vi "scripting_v4.vi"() -> ()   [LabVIEW 2020]
uses:
  <vilib>/numeric/LVNumericRepresentation.ctl
panel:
  out "appended path":path
  out "concatenated string":string
  out "resulting string":string
  out "error out 2":errorcluster
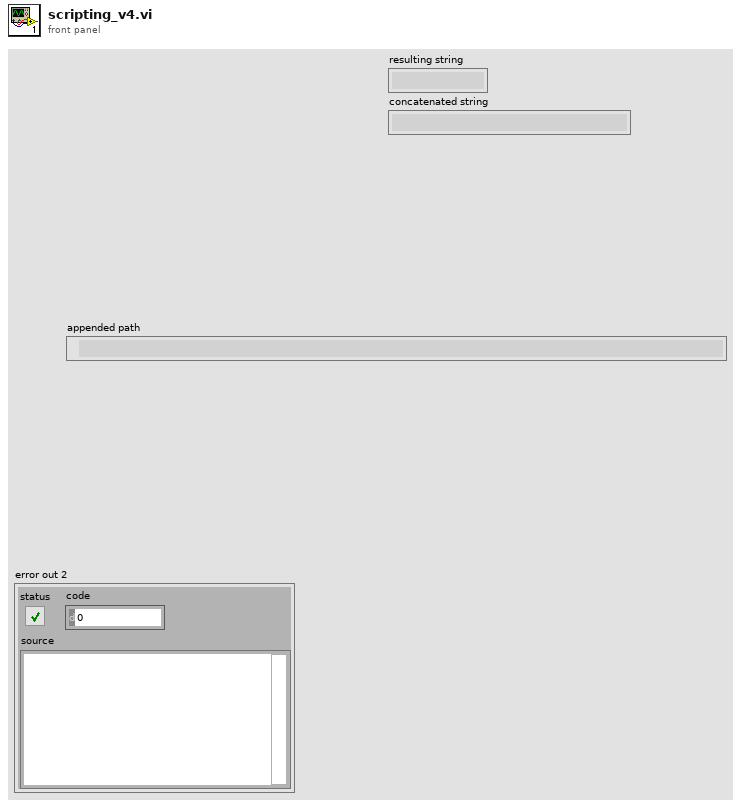
[diagram p1: front panel]
types:
  T1 = typedef "LVNumericRepresentation.ctl" = enum32{"Extended Precision", "Double Precision", "Single Precision", "Long", "Word", "Byte", "Unsigned Long", "Unsigned Word", "Unsigned Byte", "Complex Extended", "Complex Double", "Complex Single", "Quad", "Unsigned Quad", "Fixed-Point"}
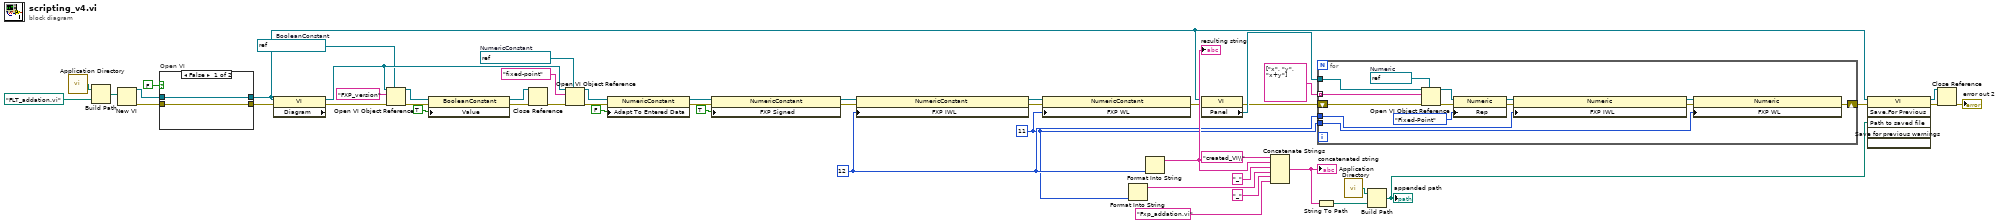
[diagram p0: block diagram]
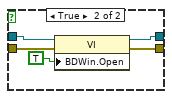
[diagram p2: hidden frame]
diagram:
  w10 = refnum<vi> refnum  # BooleanConstant
  w19 = refnum<vi> refnum  # NumericConstant
  w20 = 11 ("Fixed-Point Representation:Bits:Word Length")
  w21 = 12 ("Fixed-Point Representation:Bits:Integer Word Length")
  n1 = call <vilib>:"Application Directory.vi"() -> ("Application Directory"=w41:path)
  n2 = Build Path(base path=w41, name or relative path=path "FLT_addation.vi" ("vi path")) -> (appended path=w39:path)
  n3 = New VI(10:w39) -> (0:w49:errorcluster, 3:w50:refnum<vi>)  [unwired: 6 in]
  n4 = case "Open VI" shown="False" FALSE {
    tunnel: w50 -> [w51 w57]
    tunnel: w49 -> [w52 w56]
    tunnel: [w51 w54] -> w26
    tunnel: [w52 w53] -> w27
    frame False {
    }
    frame True {
      n5 = property class="VI"(reference=w57, error in=w56, "BDWin.Open"=TRUE ("Block Diagram Window:Open")) -> (reference out=w54:refnum<vi>, error out=w53:errorcluster)
    }
  }
  n6 = property on="Property Node" class="VI" props=["Diagram"](reference=w26, error in=w27) -> (reference out=w11:refnum<vi>, error out=w8:errorcluster)  [unwired: 1 out]
  n7 = Open VI Object Reference(7:w10, 8:w8, 10:"FXP_version" ("name/order"), 11:w11) -> (0:w6:errorcluster, 3:w7:refnum<vi>)
  n8 = property on="Property Node" class="BooleanConstant"(reference=w7, error in=w6, "Value"=TRUE ("Adapt To Entered Data")) -> (reference out=w3:refnum<vi>, error out=w2:errorcluster)
  n9 = Close Reference(reference=w3, error in (no error)=w2) -> (error out=w1:errorcluster)
  n10 = Open VI Object Reference(7:w19, 8:w1, 10:"fixed-point" ("name/order"), 11:w11) -> (0:w9:errorcluster, 3:w15:refnum<vi>)
  n11 = property on="Property Node" class="NumericConstant"(reference=w15, error in=w9, "Adapt To Entered Data"=FALSE) -> (reference out=w14:refnum<vi>, error out=w13:errorcluster)
  n12 = property on="Property Node" class="NumericConstant"(reference=w14, error in=w13, "FXP Signed"=TRUE ("Fixed-Point Representation:Bits:Signed")) -> (reference out=w18:refnum<vi>, error out=w17:errorcluster)
  n13 = property on="Property Node" class="NumericConstant"(reference=w18, error in=w17, "FXP IWL"=w21) -> (reference out=w24:refnum<vi>, error out=w23:errorcluster)
  n14 = property on="Property Node" class="NumericConstant"(reference=w24, error in=w23, "FXP WL"=w20) -> (error out=w22:errorcluster)  [unwired: 1 out]
  n15 = Format Into String(w20) -> (resulting string=w34:string)  [unwired: 3 in, 1 out]
  n16 = Format Into String(w21) -> (resulting string=w36:string)  [unwired: 3 in, 1 out]
  "resulting string" <- w36
  n17 = property on="Property Node" class="VI"(reference=w26, error in=w22) -> (error out=w43:errorcluster, "Panel"=w44:refnum<vi>)  [unwired: 1 out]
  n18 = Concatenate Strings("created_VI\\" ("string"), w36, "_" ("string"), w34, "_" ("string"), "Fxp_addation.vi" ("string")) -> (w32:string)
  "concatenated string" <- w32
  n19 = String To Path(string=w32) -> (path=w30:path)
  n20 = for {
    tunnel: w44 -> [w69]
    tunnel: w21 -> [w60]
    tunnel: w20 -> [w59]
    shift-right: [w61] -> w42
    shift-left: w43 -> [w67]
    tunnel: string[] ["x", "y", "x+y"] -> [w58] mode=indexing
    w71 = refnum<vi> refnum  # Numeric
    n21 = Open VI Object Reference(7:w71, 8:w67, 10:w58, 11:w69) -> (0:w68:errorcluster, 3:w70:refnum<vi>)
    n22 = property on="Property Node" class="Numeric"(reference=w70, error in=w68, "Rep"=LVNumericRepresentation."Fixed-Point" ("new representation")) -> (reference out=w65:refnum<vi>, error out=w64:errorcluster)
    n23 = property on="Property Node" class="Numeric"(reference=w65, error in=w64, "FXP IWL"=w60) -> (reference out=w63:refnum<vi>, error out=w62:errorcluster)
    n24 = property on="Property Node" class="Numeric"(reference=w63, error in=w62, "FXP WL"=w59) -> (error out=w61:errorcluster)  [unwired: 1 out]
  }
  n25 = call <vilib>:"Application Directory.vi"() -> ("Application Directory"=w38:path)
  n26 = Build Path(base path=w38, name or relative path=w30) -> (appended path=w37:path)
  "appended path" <- w37
  n27 = invoke class="VI" method="Save.For Previous"(reference=w26, error in=w42, "Path to saved file"=w37) -> (reference out=w48:refnum<vi>, error out=w47:errorcluster)  [unwired: 3 in, 4 out]
  n28 = Close Reference(reference=w48, error in (no error)=w47) -> (error out=→"error out 2":errorcluster)
